vi "RNG_Probe.vi"(11 "RNG":refnum<class "RNG.lvclass">) -> (2 "Value String":string, 3 "Pause VI":bool)   [LabVIEW 2020, in "OpenLvVision_OpenCv.lvlib" / "RNG.lvclass"]
uses:
  RNG.lvclass
  _LvHelpers/EdvrObject/EdvrObject.lvclass
  C:/Users/lukas/Downloads/OpenLvVision_OpenCv/SourceCode/LabView/OpenLvVision_OpenCv/_LvHelpers/EdvrObject/EdvrObject.lvclass
panel:
  out "State":u64
  out "Reference":u64 format="%.0x"
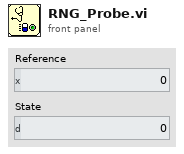
[diagram p1: front panel]
types:
  T1 = typedef "OpenLvVision_OpenCv.lvlib/EdvrObject.lvclass/Edvr.ctl" = refnum<data-value>
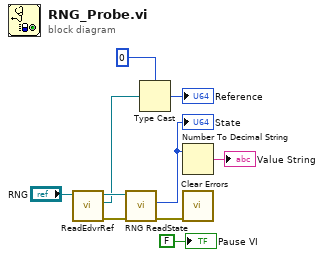
[diagram p0: block diagram]
diagram:
  n1 = call "ReadEdvrRef.vi"("EdvrObject in"="RNG") -> ("error out"=w9:errorcluster, "Edvr"=w4:T1, "EdvrObject out"=w8:refnum<class "RNG.lvclass">)  [unwired: 8 in]
  n2 = call "RNG ReadState.vi"("error in (no error)"=w9, "RNG in"=w8) -> ("error out"=w7:errorcluster, "State"=w1:u64)  [unwired: 7 in, 1 out]
  "State" <- w1
  n3 = Type Cast(type=u64 0, x=w4) -> (*(type *) &x=→"Reference":u64)
  n4 = Number To Decimal String(number=w1) -> (decimal integer string=→"Value String":string)  [unwired: 1 in]
  n5 = call <vilib>:"Clear Errors.vi"("error in (no error)"=w7) -> ()  [unwired: 5 in, 2 out]
  "Pause VI" <- FALSE
